vi "PercentDifference2.vi"(9 "percent+/-":dbl, 10 "target":dbl, 11 "achieved":dbl) -> (1 "error%":dbl format="%#_3f", 3 "closeEnough":bool)   [LabVIEW 2021]
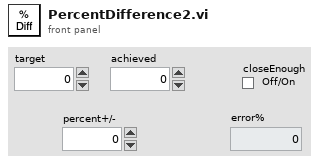
[diagram p1: front panel]
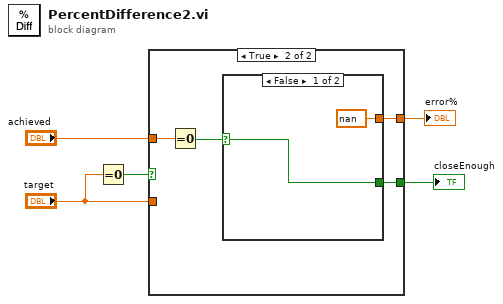
[diagram p0: block diagram]
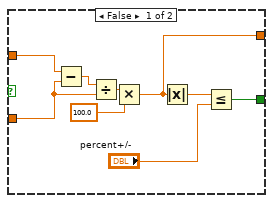
[diagram p2: hidden frame]
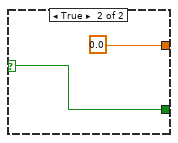
[diagram p3: hidden frame]
diagram:
  n1 = Equal To 0?(x="target") -> (x = 0?=w1:bool)
  n2 = case shown="True" w1 {
    tunnel: [w14 w15] -> w5
    tunnel: "achieved" -> [w12 w18]
    tunnel: "target" -> [w7 _]
    tunnel: [w6 w16] -> w2
    frame False {
      n3 = Subtract(x=w12, y=w7) -> (x-y=w13:dbl)
      n4 = Divide(x=w13, y=w7) -> (x/y=w10:dbl)
      n5 = Multiply(x=w10, y=100.0) -> (x*y=w6:dbl)
      n6 = Absolute Value(x=w6) -> (abs(x)=w11:dbl)
      n7 = Less Or Equal?(x=w11, y="percent+/-") -> (x <= y?=w14:bool)
    }
    frame True {
      n8 = Equal To 0?(x=w18) -> (x = 0?=w17:bool)
      n9 = case shown="False" w17 {
        selector: w17 -> [w19 w21]
        tunnel: [nan 0.0] -> w16
        tunnel: [w19 w21] -> w15
        frame False {
        }
        frame True {
        }
      }
    }
  }
  "closeEnough" <- w5
  "error%" <- w2
